vi "稱號-很大喔~.vi"() -> ()   [LabVIEW 2014]
panel:
  in  "退出視窗":bool
  # "恭喜獲得稱號:"
  # "我只能比大，不能比小"
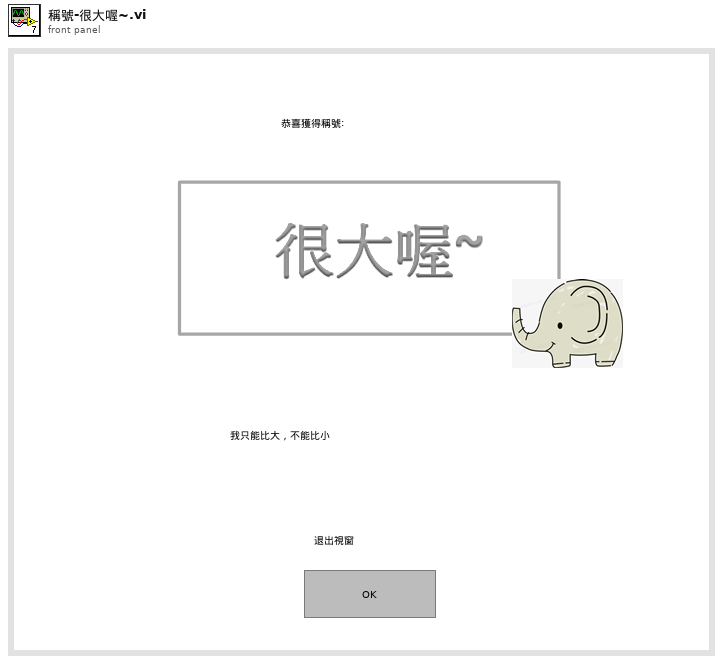
[diagram p1: front panel]
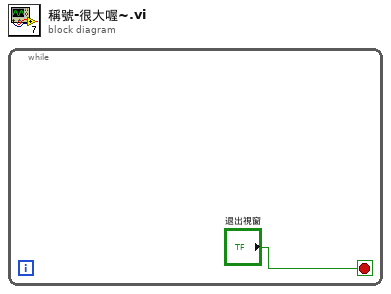
[diagram p0: block diagram]
diagram:
  n1 = while {
    stop <- "退出視窗" stop-if-true
  }
